vi "HEAVE READ.vi"(8 "error in (no error)":errorcluster, 10 "Heave and Surge Read in":string, 11 "Data Cluster":T1) -> (0 "error out":errorcluster)   [LabVIEW 2025]
uses:
  controls/LAB-IQ UI Data.ctl
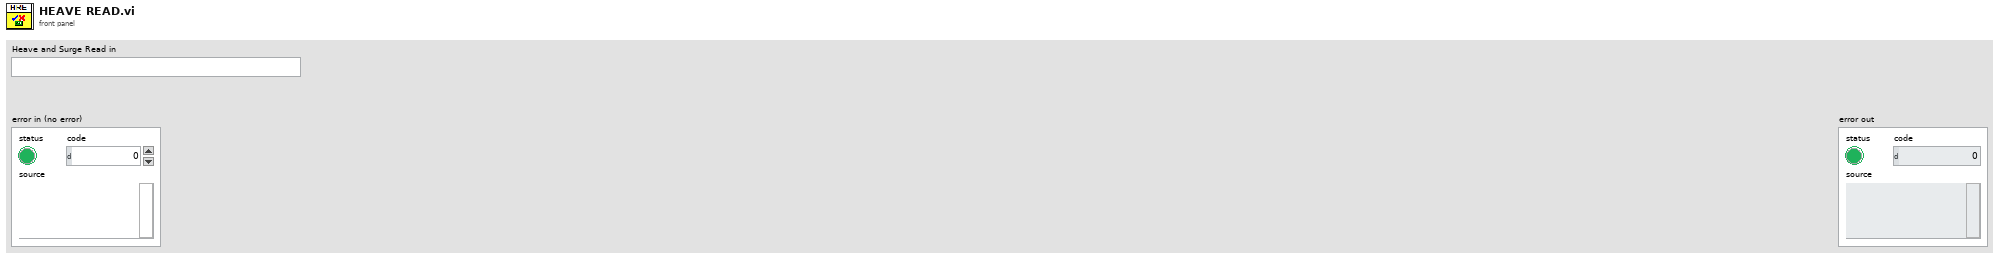
[diagram p1: front panel]
types:
  T1 = typedef "LAB-IQ UI Data.ctl" = cluster{"Main Home Screen":cluster{"GUI":refnum<vi>, "Platform Settings":refnum<vi>, "Configure":refnum<vi>, "Home":refnum<vi>, "EXIT":refnum<vi>, "service 2":refnum<vi>, "MainPage":refnum<vi>, "Analysis":refnum<vi>}, "Platform Settings":cluster{"mm/s  Surge":refnum<vi>, "Update Surge Speed":refnum<vi>, "Drive Error":refnum<vi>, "Disable Axis Jog Soft Limits":refnum<vi>, "mm/s  Sway":refnum<vi>, "Sway and Surge COM Status":refnum<vi>, "Heave COM Status":refnum<vi>, "Enable Platform":refnum<vi>, "Surge Forward Main":refnum<vi>, "Sway Right Main":refnum<vi>, "Sway Left Main":refnum<vi>, "Heave Down Main":refnum<vi>, "Heave Up main":refnum<vi>, "Update Sway Speed":refnum<vi>, "Update Heave Speed":refnum<vi>, "mm/s Heave":refnum<vi>, "mm/sec":refnum<vi>, "mm":refnum<vi>, "Surge Backward Main":refnum<vi>}, "Analysis Screen":cluster{"Analysis Home":refnum<vi>, "Surface Analysis":refnum<vi>, "Imaging":refnum<vi>, "Image Analysis":refnum<vi>, "Post Analysis":refnum<vi>}, "Config Screen":cluster{"Select Load Head":refnum<vi>, "Notes :":refnum<vi>, "FILE":refnum<vi>, "Sample ID :":refnum<vi>, "Operator ID :":refnum<vi>, "Operator Name :":refnum<vi>, "Auto":refnum<vi>}, "Motion Module":cluster{"zNL":refnum<vi>, "NL disp":refnum<vi>, "Rotary Tab":refnum<vi>, "Motion Direction:  3":refnum<vi>, "E.Velocity 2":refnum<vi>, "e.v/ssr 2":refnum<vi>, "Enter Fixed E.Velocity 2":refnum<vi>, "Enter Final SRR 2":refnum<vi>, "Enter initial SRR 2":refnum<vi>, "Enter Fixed SRR 2":refnum<vi>, "Enter the Final E.Velocity (m/s) 2":refnum<vi>, "Enter initial E.Velocity (m/s) 2":refnum<vi>, "Final Speed (RPM) 3":refnum<vi>, "Initial Speed (RPM) 2":refnum<vi>, "Enter the Final Velocity (m/s) 3":refnum<vi>, "Enter initial Velocity (m/s)  3":refnum<vi>, "Ramp Up 2":refnum<vi>, "TEST SELECTION":refnum<vi>, "SPEED SELECTION : ":refnum<vi>, "Angular Oscillation Set":refnum<vi>, "Traction":refnum<vi>, "Step Speed":refnum<vi>, "StepTable For Load-Speed":refnum<vi>, "StepTable For Speed":refnum<vi>, "Surge Forward MM":refnum<vi>, "Surge Backward MM":refnum<vi>, "M3 Image":refnum<vi>, "String 39":refnum<vi>, "Sway Left MM":refnum<vi>, "Sway Right MM":refnum<vi>, "Disable Axis Jog Soft Limits":refnum<vi>, "mm":refnum<vi>, "Heave Down MM":refnum<vi>, "Heave Up MM":refnum<vi>, "Wear Track Diameter (mm)":refnum<vi>, "Set WTD":refnum<vi>, "HomeScratch":refnum<vi>, "HomeRot":refnum<vi>, "PlaceModule":refnum<vi>, "Enter the Angle (Deg)":refnum<vi>, "Enter the Frequency (Hz)":refnum<vi>, "Motion Mode:":refnum<vi>, "LR Sway":refnum<vi>, "Rot Hor":refnum<vi>, "Scratch":refnum<vi>, "LR Cam":refnum<vi>, "MMBack":refnum<vi>, "MMNext":refnum<vi>, "Rot Ver":refnum<vi>, "Rotary Module Selection":refnum<vi>, "calculate rotary":refnum<vi>, "SPEED SELECTION : rotary":refnum<vi>, "Import 2":refnum<vi>, "Save 2":refnum<vi>, "File Path :  2":refnum<vi>, "String 45":refnum<vi>, "StepTable For Speed 3":refnum<vi>, "Enter the Speed(mm/sec)":refnum<vi>, "Enter the Speed(RPM)":refnum<vi>, "Enter Scratch Speed (mm/s):":refnum<vi>, "SwaySpeed Set":refnum<vi>, "Scartch Offset":refnum<vi>, "Motion type:":refnum<vi>, "HomeScratch 2":refnum<vi>, "Enter Scratch length (mm):":refnum<vi>, "Wear Track Diameter":refnum<vi>, "Rotary Speed Exced":refnum<vi>, "Scratch Mode":refnum<vi>, "No of Scratch":refnum<vi>}, "Environmental control":cluster{"Humidity  Status  3":refnum<vi>, "Low Temp  Status  2":refnum<vi>, "TK4 status 2":refnum<vi>, "Stage Temperature":refnum<vi>, "Sample Temperature":refnum<vi>, "Humidity (Amb)":refnum<vi>, "Clear List":refnum<vi>, "Add to list":refnum<vi>, "Wear":refnum<vi>, "Vibration":refnum<vi>, "Humidity (Chamber)":refnum<vi>, "Temperature (Chamber)":refnum<vi>, "ECR ":refnum<vi>, "Temperature (Amb)":refnum<vi>, "Microphone":refnum<vi>, "Acoustic Emission 3":refnum<vi>, "SNext":refnum<vi>, "APBack":refnum<vi>, "Enter the Temperature (°C):":refnum<vi>, "Enter the Stage \nTemperature (°C):":refnum<vi>, "Enter the Humidity (%Rh):":refnum<vi>, "Low Temp":refnum<vi>, "High Temp":refnum<vi>, "Humidity":refnum<vi>, "Sensors Picked":refnum<vi>}, "About Screen":cluster{"Password":refnum<vi>, "Home Service":refnum<vi>, "Advanced Setting":refnum<vi>, "About Tab":refnum<vi>, "ECR Port:":refnum<vi>, "Ramp Port:":refnum<vi>, "Installation/Replacement completed":refnum<vi>, "Loahead":refnum<vi>, "Heave and Surge COM Port:":refnum<vi>, "Sway COM Port:":refnum<vi>, "Temp Modbus:":refnum<vi>, "Humidity Port:":refnum<vi>, "Edit Gain Constants":refnum<vi>, "Save Gain Constants":refnum<vi>}, "Main Screen":cluster{"Main Screen Tab":refnum<vi>, "Angle and Frequency":refnum<vi>, "Stroke (mm)":refnum<vi>, "Angle (Deg)":refnum<vi>, "Main Speed Tab":refnum<vi>, "MTM MOTOR DISPLAY":refnum<vi>, "Disc Speed (m/sec)":refnum<vi>, "Ball Speed (m/sec)":refnum<vi>, "Disc Speed (RPM)":refnum<vi>, "Ball Speed (RPM)":refnum<vi>, "SPEED TAB":refnum<vi>, "Speed (m/sec)":refnum<vi>, "Set Speed (m/sec)":refnum<vi>, "Speed (RPM)":refnum<vi>, "Set Speed":refnum<vi>, "Time Tab":refnum<vi>, "Time ( HH:MM:SS ) 2":refnum<vi>, "Test Duration":refnum<vi>, "Test Duration 4":refnum<vi>, "TEST CYCLE":refnum<vi>, "TOTAL CYCLES":refnum<vi>, "Set Load (N)":refnum<vi>, "Temp Tabs":refnum<vi>, "Heater":refnum<vi>, "TK4 status":refnum<vi>, "ChamberTemp":refnum<vi>, "SetTmp":refnum<vi>, "Controller  Status":refnum<vi>, "ChamberTemp 2":refnum<vi>, "SetTmp 2":refnum<vi>, "Controller  Status 2":refnum<vi>, "ChamberTemp 3":refnum<vi>, "SetTmp 3":refnum<vi>, "Cooling":refnum<vi>, "Load Communication":refnum<vi>, "Ambient \nTemperature":refnum<vi>, "HumCOMStatus":refnum<vi>, "Ambient\n Humidity":refnum<vi>, "Freq (Hz)":refnum<vi>, "Load En":refnum<vi>, "NLt":refnum<vi>, "zNL 2":refnum<vi>, "Humidity On":refnum<vi>, "humidity disp":refnum<vi>, "Set Humidity":refnum<vi>, "NL disp 2":refnum<vi>, "Humidity On 2":refnum<vi>, "humidity disp 2":refnum<vi>, "Set Humidity 2":refnum<vi>, "NL disp 3":refnum<vi>, "AppLoadSeq scratch":refnum<vi>, "Stop Scratch":refnum<vi>, "ClrLog":refnum<vi>, "Trip Log":refnum<vi>, "STOP":refnum<vi>, "Start Test":refnum<vi>, "Test status":refnum<vi>, "AR Led":refnum<vi>, "Data":refnum<vi>, "Health":refnum<vi>, "Sway COM Status":refnum<vi>, "Heave COM Status":refnum<vi>, "Grp Tab":refnum<vi>, "Sub Graph":refnum<vi>, "SD (mm)":refnum<vi>, "Siliding distance Reset Graph":refnum<vi>, "SDGp":refnum<vi>, "Humidity Reset Graph":refnum<vi>, "HumrGp":refnum<vi>, "Acoustic Emission (mV)":refnum<vi>, "Aqucostic Reset Graph":refnum<vi>, "gACQUOS":refnum<vi>, "ECR RESET":refnum<vi>, "ECR":refnum<vi>, "Temperature Reset":refnum<vi>, "Acoustic Emission (mV) 2":refnum<vi>, "Aqucostic Reset Graph 2":refnum<vi>, "gACQUOS 2":refnum<vi>, "ECR RESET 2":refnum<vi>, "ECR 2":refnum<vi>, "Temperature Reset 2":refnum<vi>, "Temperature (deg c)":refnum<vi>, "Speed Reset Graph":refnum<vi>, "Speed Tab":refnum<vi>, "MTM DISC  SPEED":refnum<vi>, "MTM BALL SPEED":refnum<vi>, "speed mm/sec":refnum<vi>, "Hymidity":refnum<vi>, "Humidity Disable trip":refnum<vi>, "CoF Trip  2":refnum<vi>, "Depth Trip":refnum<vi>, "Weart Deapth":refnum<vi>, "Depth Reset Graph":refnum<vi>, "Weart":refnum<vi>, "Depthz":refnum<vi>, "Depth (µm)":refnum<vi>, "WearGp":refnum<vi>, "NL Trip 2":refnum<vi>, "Load pid":refnum<vi>, "Load Disable Trip":refnum<vi>, "Load Reset Graph":refnum<vi>, "NL Display 4":refnum<vi>, "Main Chart 3":refnum<vi>, "BACK":refnum<vi>, "Depth Trip 2":refnum<vi>, "COF TRIP ":refnum<vi>, "Friction Force (N)":refnum<vi>, "FF Reset Graph":refnum<vi>, "FF Disable Trip":refnum<vi>, "FF TRIP":refnum<vi>, "COF Disable Trip":refnum<vi>, "COF Reset Graph":refnum<vi>, "Start Test Temp":refnum<vi>, "zFF":refnum<vi>, "Friction Force (N) Graph":refnum<vi>, "Coefficient of Friction":refnum<vi>, "Scratch Start Test":refnum<vi>, "FF Tab":refnum<vi>, "Cyclic Friction Force (N)":refnum<vi>, "CZ FF":refnum<vi>, "Cyclic Friction Force (N) Graph":refnum<vi>, "Cyclic Coefficient of Friction":refnum<vi>, "Cyclic FF TRIP":refnum<vi>, "Cyclic FF Disable Trip":refnum<vi>, "cyclic COF Disable Trip":refnum<vi>, "cyclic COF TRIP":refnum<vi>, "cyclic COF Reset Graph":refnum<vi>, "Cyclic FF Reset Graph":refnum<vi>, "Test Trip":refnum<vi>, "Multi Scratch Pass":refnum<vi>, "Scratch Start Recording":refnum<vi>}, "Loading":cluster{"Indentation":refnum<vi>, "Reference Sample":refnum<vi>, "Load Cell Communication Slide":refnum<vi>, "com 3":refnum<vi>, "com":refnum<vi>, "DecaForce COM Status":refnum<vi>, "Update":refnum<vi>, "Clear 3":refnum<vi>, "seq":refnum<vi>, "Stribeck table":refnum<vi>, "Stribeck Table  For loading":refnum<vi>, "Loading Mode":refnum<vi>, "Enter the Final Load (N)":refnum<vi>, "Enter the CoF Trip":refnum<vi>, "Enter the Friction Force Trip":refnum<vi>, "Enter the Normal load Trip":refnum<vi>, "Enter the Load  (N)":refnum<vi>, "KiloForce":refnum<vi>, "DecaForce ":refnum<vi>, "MicroForce":refnum<vi>, "LHBack":refnum<vi>, "LHNext":refnum<vi>, "Enter the Loading Rate (N/min)":refnum<vi>, "Message":refnum<vi>, "Warning 2":refnum<vi>, "SSP 0.75":refnum<vi>, "SSP 0.5":refnum<vi>, "SSP 0.3":refnum<vi>, "Warning":refnum<vi>, "gui GIF":refnum<vi>, "Communication is established":refnum<vi>, "AppLoad 4":refnum<vi>, "Multipoint":refnum<vi>, "Load Selection":refnum<vi>}, "PID":cluster{"Ramp MulFac":refnum<vi>, "pulses LoadDiffRamp(2..10)":refnum<vi>, "PulseControlRamp(diff<=3N)":refnum<vi>, "SetLoadDeadband(%) Load(0-10N)":refnum<vi>, "PID gains out delay (microForce)":refnum<vi>, "Ramp":refnum<vi>, "Gain 2":refnum<vi>, "pulses LoadDiff(2..10)":refnum<vi>, "pulses LoadDiff(11..50)":refnum<vi>, "PulseControl(diff<=3N)":refnum<vi>, "SetLoadDeadband(%)  2":refnum<vi>, "Dummy Run":refnum<vi>, "Vertical load (N)":refnum<vi>, "AutoTune":refnum<vi>, "Offset 3 ":refnum<vi>, "apply load":refnum<vi>, "Offset  3":refnum<vi>, "apply load 2":refnum<vi>, "Enter ByPass Load":refnum<vi>, "reinit 3":refnum<vi>, "output range delay":refnum<vi>, "PID gains out delay":refnum<vi>, "Bypass Load":refnum<vi>, "pulsesSent":refnum<vi>, "pulses ":refnum<vi>, "actpid":refnum<vi>, "gFF Rot":refnum<vi>, "pulses LoadDiff(21..1000)":refnum<vi>, "Delay":refnum<vi>, "deadband":refnum<vi>}, "Config Parameters":cluster{"Tab Control 3":refnum<vi>, "Tab Control 19":refnum<vi>, "SAMPLES":refnum<vi>, "Re-initilaize":refnum<vi>, "Filter ON/OFF":refnum<vi>, "TracHomeSurgeOffsetCounts 10MM":refnum<vi>, "TracHomeSwayOffsetCounts 10MM":refnum<vi>, "Acoustic Emission:":refnum<vi>, "Apply Filter (FF)":refnum<vi>, "Filter% 2":refnum<vi>, "Apply Filter (Load)":refnum<vi>, "Filter% ":refnum<vi>, "Sway distance (mm)":refnum<vi>, "Surge distance (mm)":refnum<vi>, "DataSavingLoopDelay(ms)":refnum<vi>, "SAVE 2":refnum<vi>, "Enter Distance":refnum<vi>, "Sway Counts:":refnum<vi>, "Distance (mm): 3":refnum<vi>, "Surge Counts:":refnum<vi>, "Distance (mm): 2":refnum<vi>, "Distance (mm):":refnum<vi>, "Heave Counts:":refnum<vi>, "LRMHomeSurgeOffsetCounts":refnum<vi>, "LRMHomeSwayOffsetCounts":refnum<vi>, "TracHomeSurgeOffsetCounts 20MM":refnum<vi>, "TracHomeSwayOffsetCounts 20MM":refnum<vi>, "RotHomeSwayOffsetCounts":refnum<vi>, "RotHomeSurgeOffsetCounts":refnum<vi>, "Heave distance":refnum<vi>, "Zmm":refnum<vi>, "Heave Pulses/mm":refnum<vi>, "Surge Pulses/mm":refnum<vi>, "Sway Pulses/mm":refnum<vi>, "Heave Pitch":refnum<vi>, "Surge Pitch":refnum<vi>, "Sway Pitch":refnum<vi>, "Heave PPR":refnum<vi>, "Surge PPR":refnum<vi>, "Sway PPR":refnum<vi>, "Tab Control 5":refnum<vi>, "Tab Control 14":refnum<vi>, "Tab Control 26":refnum<vi>, "AE":refnum<vi>, "Heave Loop Delay":refnum<vi>, "Heave PID Speed":refnum<vi>, "Surge Jog Speed":refnum<vi>, "Heave Jog Speed":refnum<vi>, "Sway Loop Delay":refnum<vi>, "Sway PID Speed":refnum<vi>, "Sway Jog Speed":refnum<vi>, "DEPTH TRIP VALUE":refnum<vi>, "LOAD TRIP VALUE":refnum<vi>, "DEPTH TRIP   ENABLE":refnum<vi>, "LOAD TRIP  ENABLE":refnum<vi>, "CYCLIC FF TRIP VALUE":refnum<vi>, "FF TRIP VALUE":refnum<vi>, "CYCLIC CoF TRIP VALUE":refnum<vi>, "COF TRIP VALUE":refnum<vi>, "CYCLIC COF TRIP  ENABLE":refnum<vi>, "CYCLIC FF TRIP  ENABLE":refnum<vi>, "FF TRIP  ENABLE":refnum<vi>, "COF TRIP  ENABLE":refnum<vi>}, "Loading Com Port":cluster{"ClearAll":refnum<vi>, "Mz(Nm)":refnum<vi>, "My(Nm)":refnum<vi>, "Mx(Nm)":refnum<vi>, "Save Dwell":refnum<vi>, "Mx ":refnum<vi>, "My ":refnum<vi>, "Mz":refnum<vi>, "Fx(N)":refnum<vi>, "Fy(N)":refnum<vi>, "Fz(N)":refnum<vi>, "ZeroAll":refnum<vi>, "Acq Delay (ms)":refnum<vi>, "Burst Delay (ms)":refnum<vi>, "model":refnum<vi>, "SN":refnum<vi>, "FFx(N)":refnum<vi>, "Sensor IP":refnum<vi>, "Port":refnum<vi>, "FFy(N)":refnum<vi>, "Load(N)":refnum<vi>, "delete Handle":refnum<vi>, "Create Handle":refnum<vi>, "ft_data":refnum<vi>, "ft_range":refnum<vi>, "ft_data 2":refnum<vi>, "stop 6":refnum<vi>, "running_flag":refnum<vi>, "ft_udp_handle":refnum<vi>, "get-data-return":refnum<vi>, "get-range-return":refnum<vi>, "zero-return":refnum<vi>, "filter-return":refnum<vi>, "initial-return":refnum<vi>, "deleteHandle-result":refnum<vi>, "Load Cell Temp":refnum<vi>}, "Heave AND Surge":cluster{"SURGE POSE":refnum<vi>, "error out Read":refnum<vi>, "HEAVE POSE":refnum<vi>, "State":refnum<vi>, "Homed":refnum<vi>, "Sequence ID":refnum<vi>, "error out Write":refnum<vi>, "faultCode":refnum<vi>, "Ack ID":refnum<vi>, "SPEED":refnum<vi>, "Distance":refnum<vi>, "Mode Command":refnum<vi>, "Heave and Surge Read":refnum<vi>, "Read Heave Temp":refnum<vi>, "Spare 15":refnum<vi>, "Spare 14":refnum<vi>, "Spare 13":refnum<vi>, "Spare 12":refnum<vi>, "Spare 11":refnum<vi>, "Spare 10":refnum<vi>, "Spare 9":refnum<vi>, "Spare 8":refnum<vi>, "Spare 7":refnum<vi>, "Spare 6":refnum<vi>, "Spare 5":refnum<vi>, "Spare 4":refnum<vi>, "Spare 2":refnum<vi>, "Spare 1":refnum<vi>, "Node Id":refnum<vi>, "Spare 3":refnum<vi>, "SPARE 4":refnum<vi>, "SPARE 3":refnum<vi>, "SPARE 2":refnum<vi>, "SPARE 1":refnum<vi>, "fwMajor":refnum<vi>, "fwMinor":refnum<vi>, "Manual Write":refnum<vi>, "Heave and Surge Write":refnum<vi>}, "New PID LOGIC":cluster{"Fine Tune Zone":refnum<vi>, "PID SDelay":refnum<vi>, "Max_pos_limit":refnum<vi>, "Min_pos_limit":refnum<vi>, "i_limit":refnum<vi>, "pct_scale":refnum<vi>, "Deadband":refnum<vi>, "Kd":refnum<vi>, "Ki":refnum<vi>, "Kp":refnum<vi>, "Current Position":refnum<vi>, "Set Load":refnum<vi>, "Current Load":refnum<vi>, "Pulse delta":refnum<vi>, "Init Step":refnum<vi>, "Max Step Linit":refnum<vi>}, "SWAY ":cluster{"fwMajor":refnum<vi>, "Homed":refnum<vi>, "Rotary POSE":refnum<vi>, "State":refnum<vi>, "SWAY POSE":refnum<vi>, "Ack ID":refnum<vi>, "faultCode":refnum<vi>, "Node Id":refnum<vi>, "fwMinor":refnum<vi>, "Spare 6":refnum<vi>, "Spare 5":refnum<vi>, "Spare 4":refnum<vi>, "Spare 3":refnum<vi>, "Spare 2":refnum<vi>, "Spare 1":refnum<vi>, "Spare 7":refnum<vi>, "SPARE  5":refnum<vi>, "error out Write  SWAY ":refnum<vi>, "error out Read SWAY ":refnum<vi>, "Manual Write SWAY ":refnum<vi>, "SWAY WRITE":refnum<vi>, "SPARE  4":refnum<vi>, "SPARE  3":refnum<vi>, "SPARE 2":refnum<vi>, "SPARE 1":refnum<vi>, "Spare 15":refnum<vi>, "Spare 14":refnum<vi>, "Spare 13":refnum<vi>, "Spare 12":refnum<vi>, "Spare 11":refnum<vi>, "Spare 9":refnum<vi>, "Spare 8":refnum<vi>, "SPEED":refnum<vi>, "Distance":refnum<vi>, "Mode Command":refnum<vi>, "Sequence ID":refnum<vi>, "SWAY READ":refnum<vi>, "Spare 10":refnum<vi>, "Read SWAY Temp":refnum<vi>}, "Analysis Screen":cluster{"Analysis Home":refnum<vi>, "Refresh 2":refnum<vi>, "MEAN 4":refnum<vi>, "SD 4":refnum<vi>, "VARIANCE 4":refnum<vi>, "MEAN  3":refnum<vi>, "SD  3":refnum<vi>, "VARIANCE  3":refnum<vi>, "MEAN 2":refnum<vi>, "SD  2":refnum<vi>, "VARIANCE 2":refnum<vi>, "MEAN":refnum<vi>, "SD":refnum<vi>, "VARIANCE":refnum<vi>, "File 4 Discription":refnum<vi>, "OPEN 4":refnum<vi>, "File Name 4":refnum<vi>, "OPEN 3":refnum<vi>, "File 3 Discription":refnum<vi>, "File Name 3":refnum<vi>, "Y-AXIS":refnum<vi>, "X-AXIS":refnum<vi>, "XY Graph":refnum<vi>, "File Name 2":refnum<vi>, "File Name 1":refnum<vi>, "OPEN 2":refnum<vi>, "OPEN 1":refnum<vi>, "File 1 Discription ":refnum<vi>, "File 2 Discription":refnum<vi>, "Export":refnum<vi>, "File Format":refnum<vi>}}
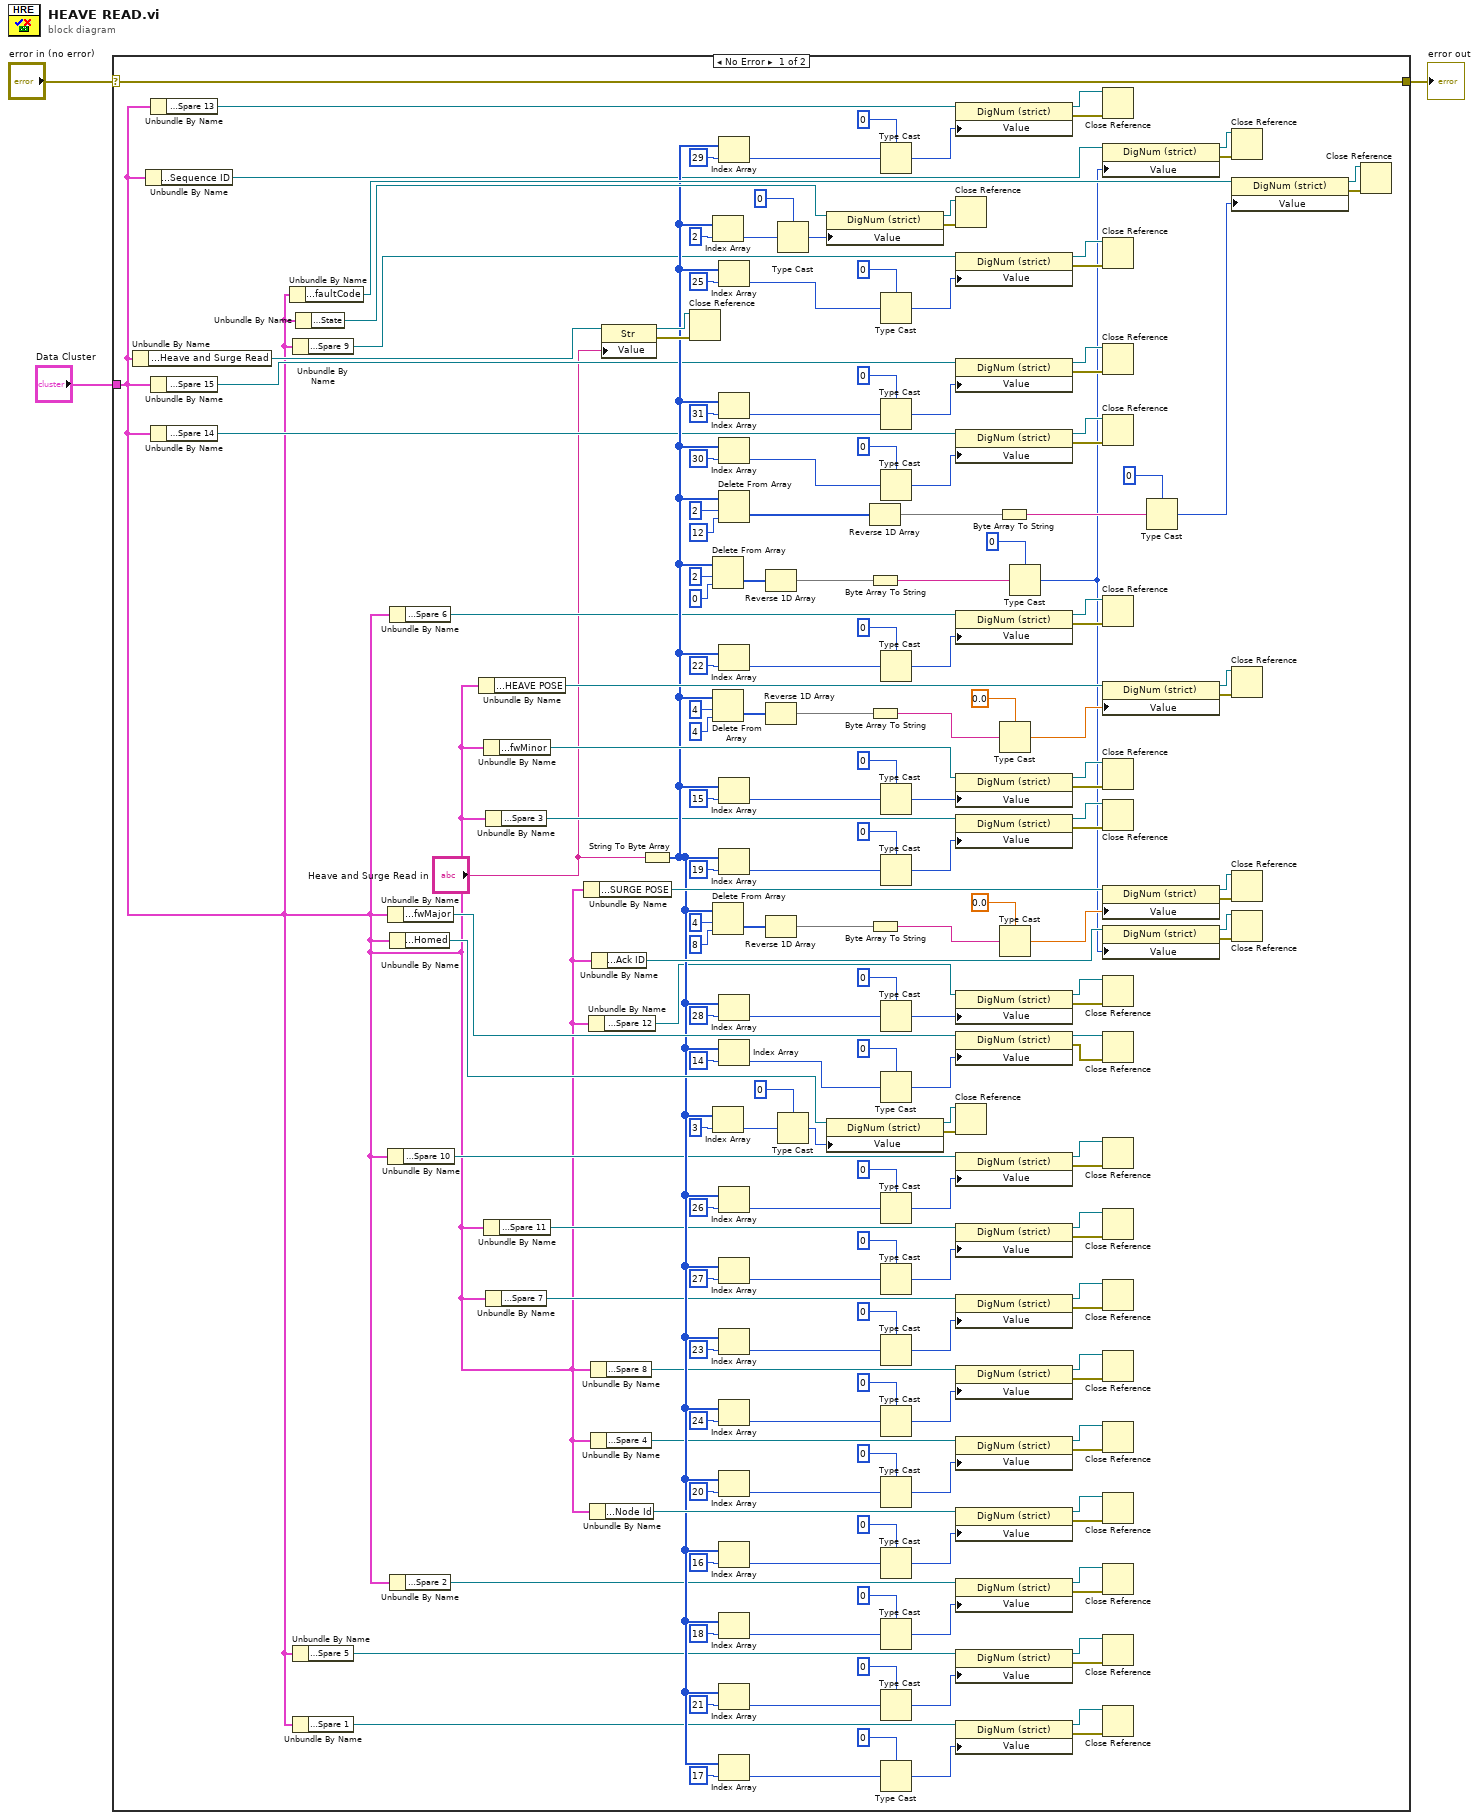
[diagram p0: block diagram]
diagram:
  n1 = case shown="No Error" "error in (no error)" {
    selector: "error in (no error)" -> [w5 _]
    tunnel: "Data Cluster" -> [w6 _]
    tunnel: [w5 _] -> w3
    frame No Error {
      n2 = Unbundle By Name(w6) -> ("Heave AND Surge.Heave and Surge Read"=w193:refnum<vi>)
      n3 = Unbundle By Name(w6) -> ("Heave AND Surge.Sequence ID"=w9:refnum<vi>)
      n4 = Unbundle By Name(w6) -> ("Heave AND Surge.Spare 13"=w38:refnum<vi>)
      n5 = Unbundle By Name(w6) -> ("Heave AND Surge.Spare 15"=w30:refnum<vi>)
      n6 = Unbundle By Name(w6) -> ("Heave AND Surge.Spare 14"=w33:refnum<vi>)
      n7 = Unbundle By Name(w6) -> ("Heave AND Surge.faultCode"=w132:refnum<vi>)
      n8 = Unbundle By Name(w6) -> ("Heave AND Surge.Spare 9"=w18:refnum<vi>)
      n9 = Unbundle By Name(w6) -> ("Heave AND Surge.Spare 5"=w47:refnum<vi>)
      n10 = Unbundle By Name(w6) -> ("Heave AND Surge.Spare 1"=w70:refnum<vi>)
      n11 = Unbundle By Name(w6) -> ("Heave AND Surge.State"=w147:refnum<vi>)
      n12 = Unbundle By Name(w6) -> ("Heave AND Surge.fwMajor"=w126:refnum<vi>)
      n13 = Unbundle By Name(w6) -> ("Heave AND Surge.Spare 10"=w23:refnum<vi>)
      n14 = Unbundle By Name(w6) -> ("Heave AND Surge.Spare 6"=w52:refnum<vi>)
      n15 = Unbundle By Name(w6) -> ("Heave AND Surge.Homed"=w143:refnum<vi>)
      n16 = Unbundle By Name(w6) -> ("Heave AND Surge.Spare 2"=w65:refnum<vi>)
      n17 = Unbundle By Name(w6) -> ("Heave AND Surge.HEAVE POSE"=w140:refnum<vi>)
      n18 = Unbundle By Name(w6) -> ("Heave AND Surge.fwMinor"=w122:refnum<vi>)
      n19 = Unbundle By Name(w6) -> ("Heave AND Surge.Spare 11"=w29:refnum<vi>)
      n20 = Unbundle By Name(w6) -> ("Heave AND Surge.Spare 3"=w59:refnum<vi>)
      n21 = Unbundle By Name(w6) -> ("Heave AND Surge.Spare 7"=w58:refnum<vi>)
      n22 = Unbundle By Name(w6) -> ("Heave AND Surge.SURGE POSE"=w134:refnum<vi>)
      n23 = Unbundle By Name(w6) -> ("Heave AND Surge.Spare 12"=w24:refnum<vi>)
      n24 = Unbundle By Name(w6) -> ("Heave AND Surge.Node Id"=w118:refnum<vi>)
      n25 = Unbundle By Name(w6) -> ("Heave AND Surge.Spare 8"=w53:refnum<vi>)
      n26 = Unbundle By Name(w6) -> ("Heave AND Surge.Spare 4"=w64:refnum<vi>)
      n27 = Unbundle By Name(w6) -> ("Heave AND Surge.Ack ID"=w150:refnum<vi>)
      n28 = property class="Str"(reference=w193, "Value"="Heave and Surge Read in") -> (reference out=w191:refnum<vi>, error out=w192:errorcluster)  [unwired: 1 in]
      n29 = String To Byte Array(string="Heave and Surge Read in") -> (unsigned byte array=w71:u8[])
      n30 = Close Reference(reference=w191, error in (no error)=w192) -> ()  [unwired: 1 out]
      n31 = Index Array(array=w71, index=2) -> (element=w183:u8)
      n32 = Delete From Array(array=w71, length=2, index=0) -> (deleted portion=w157:u8[])  [unwired: 1 out]
      n33 = Delete From Array(array=w71, length=4, index=4) -> (deleted portion=w155:u8[])  [unwired: 1 out]
      n34 = Delete From Array(array=w71, length=4, index=8) -> (deleted portion=w158:u8[])  [unwired: 1 out]
      n35 = Index Array(array=w71, index=3) -> (element=w182:u8)
      n36 = Index Array(array=w71, index=29) -> (element=w74:u8)
      n37 = Index Array(array=w71, index=25) -> (element=w90:u8)
      n38 = Index Array(array=w71, index=31) -> (element=w78:u8)
      n39 = Index Array(array=w71, index=30) -> (element=w75:u8)
      n40 = Delete From Array(array=w71, length=2, index=12) -> (deleted portion=w156:u8[])  [unwired: 1 out]
      n41 = Index Array(array=w71, index=22) -> (element=w96:u8)
      n42 = Index Array(array=w71, index=15) -> (element=w159:u8)
      n43 = Index Array(array=w71, index=19) -> (element=w107:u8)
      n44 = Index Array(array=w71, index=28) -> (element=w84:u8)
      n45 = Index Array(array=w71, index=14) -> (element=w161:u8)
      n46 = Index Array(array=w71, index=26) -> (element=w89:u8)
      n47 = Index Array(array=w71, index=27) -> (element=w83:u8)
      n48 = Index Array(array=w71, index=23) -> (element=w102:u8)
      n49 = Index Array(array=w71, index=24) -> (element=w101:u8)
      n50 = Index Array(array=w71, index=20) -> (element=w108:u8)
      n51 = Index Array(array=w71, index=16) -> (element=w154:u8)
      n52 = Index Array(array=w71, index=18) -> (element=w113:u8)
      n53 = Index Array(array=w71, index=21) -> (element=w95:u8)
      n54 = Index Array(array=w71, index=17) -> (element=w114:u8)
      n55 = Reverse 1D Array(array=w157) -> (reversed array=w188:u8[])
      n56 = Reverse 1D Array(array=w155) -> (reversed array=w177:u8[])
      n57 = Reverse 1D Array(array=w158) -> (reversed array=w173:u8[])
      n58 = Type Cast(type=u8 0, x=w183) -> (*(type *) &x=w145:u8)
      n59 = Type Cast(type=u8 0, x=w182) -> (*(type *) &x=w141:u8)
      n60 = property class="DigNum (strict)"(reference=w147, "Value"=w145) -> (reference out=w148:refnum<vi>, error out=w146:errorcluster)  [unwired: 1 in]
      n61 = property class="DigNum (strict)"(reference=w143, "Value"=w141) -> (reference out=w142:refnum<vi>, error out=w144:errorcluster)  [unwired: 1 in]
      n62 = Reverse 1D Array(array=w156) -> (reversed array=w167:u8[])
      n63 = Byte Array To String(unsigned byte array=w188) -> (string=w186:string)
      n64 = Byte Array To String(unsigned byte array=w177) -> (string=w175:string)
      n65 = Byte Array To String(unsigned byte array=w173) -> (string=w174:string)
      n66 = Type Cast(type=u8 0, x=w74) -> (*(type *) &x=w13:u8)
      n67 = Type Cast(type=u8 0, x=w90) -> (*(type *) &x=w17:u8)
      n68 = Type Cast(type=u8 0, x=w78) -> (*(type *) &x=w11:u8)
      n69 = Type Cast(type=u8 0, x=w75) -> (*(type *) &x=w12:u8)
      n70 = Type Cast(type=u8 0, x=w96) -> (*(type *) &x=w41:u8)
      n71 = Type Cast(type=u8 0, x=w159) -> (*(type *) &x=w121:u8)
      n72 = Type Cast(type=u8 0, x=w107) -> (*(type *) &x=w44:u8)
      n73 = Type Cast(type=u8 0, x=w84) -> (*(type *) &x=w14:u8)
      n74 = Type Cast(type=u8 0, x=w161) -> (*(type *) &x=w125:u8)
      n75 = Type Cast(type=u8 0, x=w89) -> (*(type *) &x=w16:u8)
      n76 = Type Cast(type=u8 0, x=w83) -> (*(type *) &x=w15:u8)
      n77 = Type Cast(type=u8 0, x=w102) -> (*(type *) &x=w40:u8)
      n78 = Type Cast(type=u8 0, x=w101) -> (*(type *) &x=w39:u8)
      n79 = Type Cast(type=u8 0, x=w108) -> (*(type *) &x=w43:u8)
      n80 = Type Cast(type=u8 0, x=w154) -> (*(type *) &x=w117:u8)
      n81 = Type Cast(type=u8 0, x=w113) -> (*(type *) &x=w45:u8)
      n82 = Type Cast(type=u8 0, x=w95) -> (*(type *) &x=w42:u8)
      n83 = Type Cast(type=u8 0, x=w114) -> (*(type *) &x=w46:u8)
      n84 = property class="DigNum (strict)"(reference=w38, "Value"=w13) -> (reference out=w36:refnum<vi>, error out=w37:errorcluster)  [unwired: 1 in]
      n85 = Close Reference(reference=w148, error in (no error)=w146) -> ()  [unwired: 1 out]
      n86 = property class="DigNum (strict)"(reference=w18, "Value"=w17) -> (reference out=w20:refnum<vi>, error out=w19:errorcluster)  [unwired: 1 in]
      n87 = property class="DigNum (strict)"(reference=w30, "Value"=w11) -> (reference out=w32:refnum<vi>, error out=w31:errorcluster)  [unwired: 1 in]
      n88 = property class="DigNum (strict)"(reference=w33, "Value"=w12) -> (reference out=w35:refnum<vi>, error out=w34:errorcluster)  [unwired: 1 in]
      n89 = property class="DigNum (strict)"(reference=w52, "Value"=w41) -> (reference out=w50:refnum<vi>, error out=w51:errorcluster)  [unwired: 1 in]
      n90 = property class="DigNum (strict)"(reference=w122, "Value"=w121) -> (reference out=w124:refnum<vi>, error out=w123:errorcluster)  [unwired: 1 in]
      n91 = property class="DigNum (strict)"(reference=w59, "Value"=w44) -> (reference out=w61:refnum<vi>, error out=w60:errorcluster)  [unwired: 1 in]
      n92 = property class="DigNum (strict)"(reference=w24, "Value"=w14) -> (reference out=w26:refnum<vi>, error out=w25:errorcluster)  [unwired: 1 in]
      n93 = property class="DigNum (strict)"(reference=w126, "Value"=w125) -> (reference out=w128:refnum<vi>, error out=w127:errorcluster)  [unwired: 1 in]
      n94 = Close Reference(reference=w142, error in (no error)=w144) -> ()  [unwired: 1 out]
      n95 = property class="DigNum (strict)"(reference=w23, "Value"=w16) -> (reference out=w21:refnum<vi>, error out=w22:errorcluster)  [unwired: 1 in]
      n96 = property class="DigNum (strict)"(reference=w29, "Value"=w15) -> (reference out=w27:refnum<vi>, error out=w28:errorcluster)  [unwired: 1 in]
      n97 = property class="DigNum (strict)"(reference=w58, "Value"=w40) -> (reference out=w56:refnum<vi>, error out=w57:errorcluster)  [unwired: 1 in]
      n98 = property class="DigNum (strict)"(reference=w53, "Value"=w39) -> (reference out=w55:refnum<vi>, error out=w54:errorcluster)  [unwired: 1 in]
      n99 = property class="DigNum (strict)"(reference=w64, "Value"=w43) -> (reference out=w62:refnum<vi>, error out=w63:errorcluster)  [unwired: 1 in]
      n100 = property class="DigNum (strict)"(reference=w118, "Value"=w117) -> (reference out=w120:refnum<vi>, error out=w119:errorcluster)  [unwired: 1 in]
      n101 = property class="DigNum (strict)"(reference=w65, "Value"=w45) -> (reference out=w67:refnum<vi>, error out=w66:errorcluster)  [unwired: 1 in]
      n102 = property class="DigNum (strict)"(reference=w47, "Value"=w42) -> (reference out=w49:refnum<vi>, error out=w48:errorcluster)  [unwired: 1 in]
      n103 = property class="DigNum (strict)"(reference=w70, "Value"=w46) -> (reference out=w68:refnum<vi>, error out=w69:errorcluster)  [unwired: 1 in]
      n104 = Byte Array To String(unsigned byte array=w167) -> (string=w166:string)
      n105 = Type Cast(type=sgl 0.0, x=w175) -> (*(type *) &x=w138:sgl)
      n106 = Type Cast(type=sgl 0.0, x=w174) -> (*(type *) &x=w133:sgl)
      n107 = Type Cast(type=u16 0, x=w186) -> (*(type *) &x=w7:u16)
      n108 = Close Reference(reference=w36, error in (no error)=w37) -> ()  [unwired: 1 out]
      n109 = property class="DigNum (strict)"(reference=w9, "Value"=w7) -> (reference out=w10:refnum<vi>, error out=w8:errorcluster)  [unwired: 1 in]
      n110 = Close Reference(reference=w20, error in (no error)=w19) -> ()  [unwired: 1 out]
      n111 = Close Reference(reference=w32, error in (no error)=w31) -> ()  [unwired: 1 out]
      n112 = Close Reference(reference=w35, error in (no error)=w34) -> ()  [unwired: 1 out]
      n113 = Close Reference(reference=w50, error in (no error)=w51) -> ()  [unwired: 1 out]
      n114 = property class="DigNum (strict)"(reference=w140, "Value"=w138) -> (reference out=w137:refnum<vi>, error out=w139:errorcluster)  [unwired: 1 in]
      n115 = Close Reference(reference=w124, error in (no error)=w123) -> ()  [unwired: 1 out]
      n116 = Close Reference(reference=w61, error in (no error)=w60) -> ()  [unwired: 1 out]
      n117 = property class="DigNum (strict)"(reference=w134, "Value"=w133) -> (reference out=w136:refnum<vi>, error out=w135:errorcluster)  [unwired: 1 in]
      n118 = property class="DigNum (strict)"(reference=w150, "Value"=w7) -> (reference out=w149:refnum<vi>, error out=w151:errorcluster)  [unwired: 1 in]
      n119 = Close Reference(reference=w26, error in (no error)=w25) -> ()  [unwired: 1 out]
      n120 = Close Reference(reference=w128, error in (no error)=w127) -> ()  [unwired: 1 out]
      n121 = Close Reference(reference=w21, error in (no error)=w22) -> ()  [unwired: 1 out]
      n122 = Close Reference(reference=w27, error in (no error)=w28) -> ()  [unwired: 1 out]
      n123 = Close Reference(reference=w56, error in (no error)=w57) -> ()  [unwired: 1 out]
      n124 = Close Reference(reference=w55, error in (no error)=w54) -> ()  [unwired: 1 out]
      n125 = Close Reference(reference=w62, error in (no error)=w63) -> ()  [unwired: 1 out]
      n126 = Close Reference(reference=w120, error in (no error)=w119) -> ()  [unwired: 1 out]
      n127 = Close Reference(reference=w67, error in (no error)=w66) -> ()  [unwired: 1 out]
      n128 = Close Reference(reference=w49, error in (no error)=w48) -> ()  [unwired: 1 out]
      n129 = Close Reference(reference=w68, error in (no error)=w69) -> ()  [unwired: 1 out]
      n130 = Type Cast(type=u16 0, x=w166) -> (*(type *) &x=w129:u16)
      n131 = Close Reference(reference=w10, error in (no error)=w8) -> ()  [unwired: 1 out]
      n132 = property class="DigNum (strict)"(reference=w132, "Value"=w129) -> (reference out=w130:refnum<vi>, error out=w131:errorcluster)  [unwired: 1 in]
      n133 = Close Reference(reference=w137, error in (no error)=w139) -> ()  [unwired: 1 out]
      n134 = Close Reference(reference=w136, error in (no error)=w135) -> ()  [unwired: 1 out]
      n135 = Close Reference(reference=w149, error in (no error)=w151) -> ()  [unwired: 1 out]
      n136 = Close Reference(reference=w130, error in (no error)=w131) -> ()  [unwired: 1 out]
    }
    frame Error {
    }
  }
  "error out" <- w3
